vi "hi_cur.vi"(11 "file path":path=path "C:/luminartech/ManufacturingTools/TS_Automation/Programs/Labview/bring_up/hi_cur/hi_cur_resp.txt") -> (3 "opt_power":i32)   [LabVIEW 2018]
panel:
  out "text":string
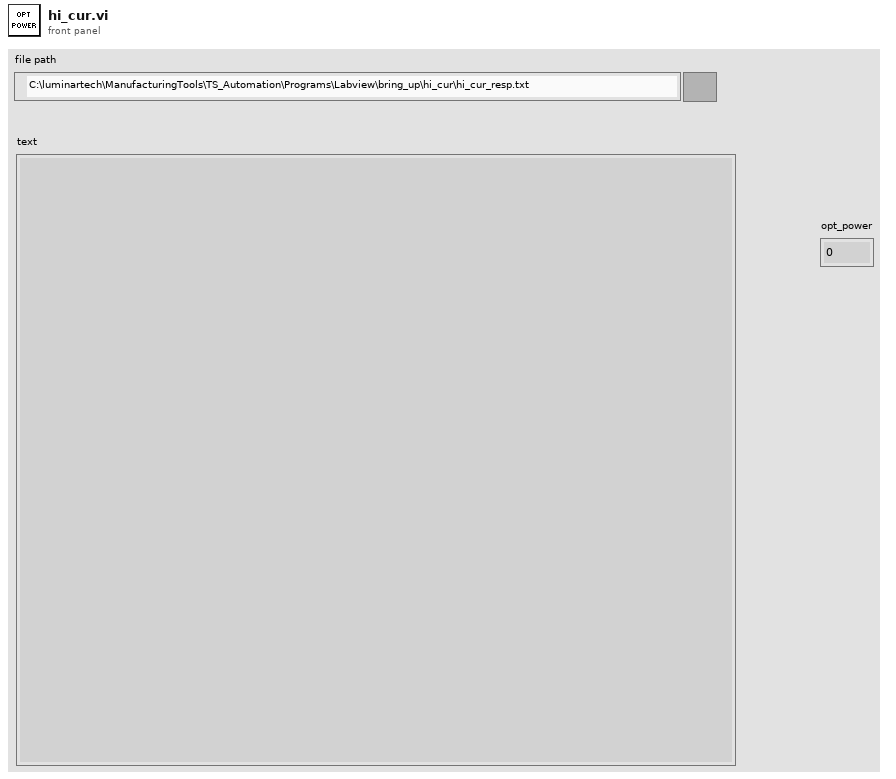
[diagram p1: front panel]
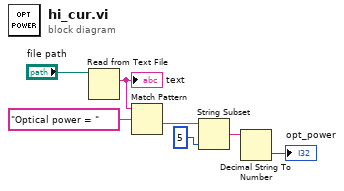
[diagram p0: block diagram]
diagram:
  n1 = Read from Text File(file (use dialog)="file path") -> (text=w4:string)  [unwired: 3 in, 3 out]
  "text" <- w4
  n2 = Match Pattern(string=w4, regular expression="Optical power = ") -> (after substring=w3:string)  [unwired: 1 in, 3 out]
  n3 = String Subset(string=w3, length (rest)=5 ("length (rest)")) -> (substring=w2:string)  [unwired: 1 in]
  n4 = Decimal String To Number(string=w2) -> (number=→"opt_power":i32)  [unwired: 2 in, 1 out]
